vi "read.vi"(8 "error in (no error)":errorcluster, 10 "block size":i32, 11 "SignalReader in":refnum<class "GenericSignalReader.lvclass">) -> (0 "error out":errorcluster, 1 "finished?":bool, 2 "signals read":dbl[][](array[numeric]), 3 "SignalReader out":refnum<class "GenericSignalReader.lvclass">, 4 "buffer overflow?":bool)   [LabVIEW 2010, in "GenericSignalReader.lvclass"]
uses:
  GenericSignalReader.lvclass
  GenericSignalReader.lvclass/GenericSignalReader.ctl
  common/classes/GenericComponent/GenericComponent/class_data.vi
  common/classes/GenericComponent/GenericComponent/GenericComponent.lvclass
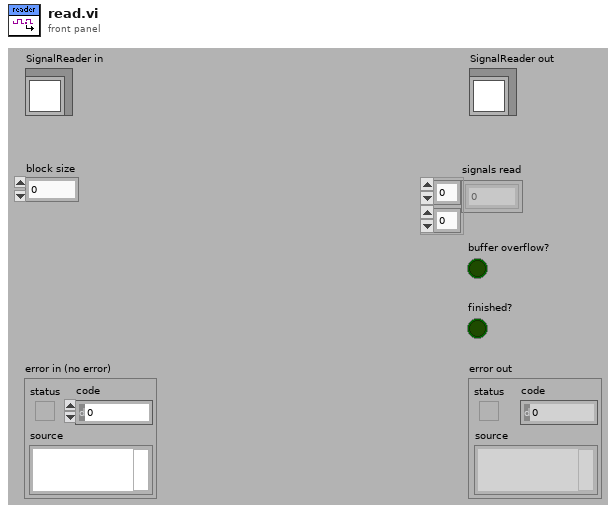
[diagram p1: front panel]
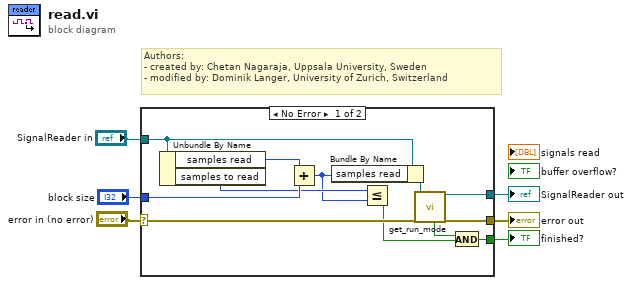
[diagram p0: block diagram]
diagram:
  # "Authors: \n- created by: Chetan Nagaraja, Uppsala University, Sweden\n- modified by: Dominik Langer, University of Zurich, Switzerland"
  n1 = case shown="No Error" "error in (no error)" {
    selector: "error in (no error)" -> [w13 w20]
    tunnel: [w12 w20] -> w5
    tunnel: [w10 w19] -> w3
    tunnel: "SignalReader in" -> [w18 w19]
    tunnel: "block size" -> [w16 _]
    tunnel: [w7 _] -> w1
    frame No Error {
      n2 = Unbundle By Name(w18) -> ("samples read"=w17:i32, "samples to read"=w15:i32)
      n3 = Add(x=w17, y=w16) -> (x+y=w14:i32)
      n4 = Bundle By Name(cluster=w18, "samples read"=w14) -> (w11:refnum<class "GenericSignalReader.lvclass">)
      n5 = Less Or Equal?(x=w15, y=w14) -> (x <= y?=w8:bool)
      n6 = call "get_run_mode.vi"("error in (no error)"=w13, "GenericPlugin in"=w11) -> ("error out"=w12:errorcluster, "GenericPlugin out"=w10:refnum<class "GenericSignalReader.lvclass">, "is NOT free run?"=w9:bool)  [unwired: 5 in, 2 out]
      n7 = And(x=w9, y=w8) -> (x .and. y?=w7:bool)
    }
    frame Error {
    }
  }
  "error out" <- w5
  "SignalReader out" <- w3
  "finished?" <- w1
